vi "CPU_MEM_read_mem.vi"(11 "address":u16 format="%04x") -> (3 "value out":u8 format="%02x")   [LabVIEW 2018]
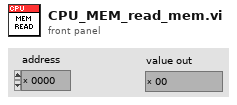
[diagram p1: front panel]
types:
  T1 = enum16{"init", "read DDR", "read PDR", "write DDR", "write PDR"}
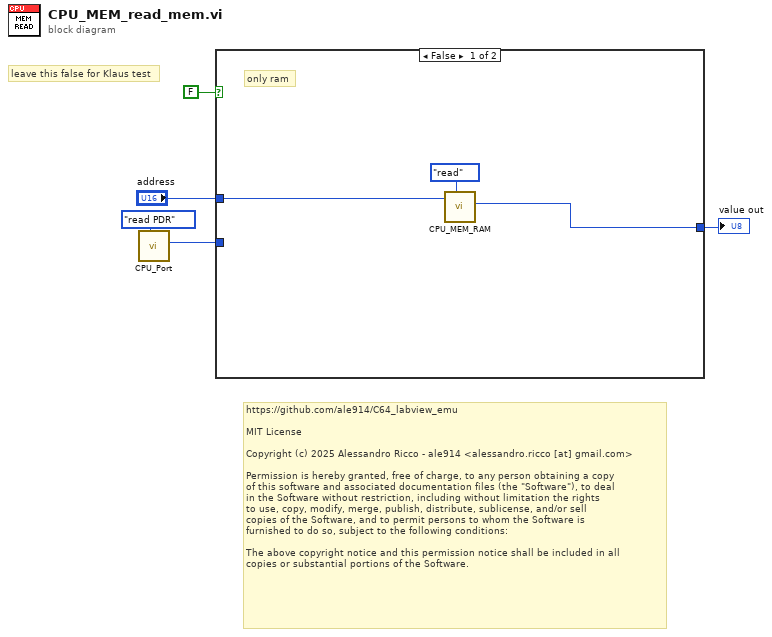
[diagram p0: block diagram]
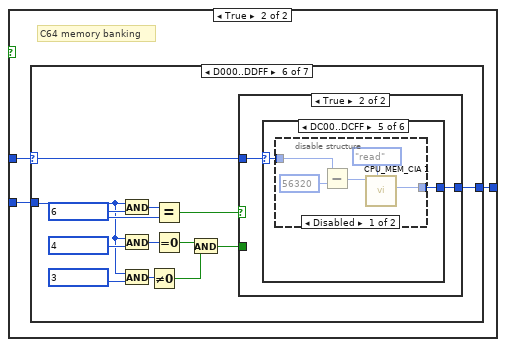
[diagram p2: hidden frame]
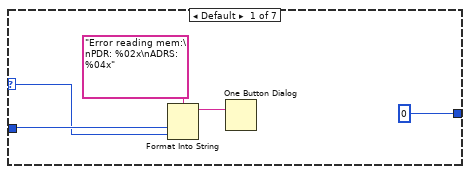
[diagram p3: hidden frame]
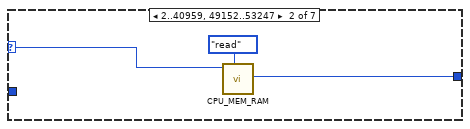
[diagram p4: hidden frame]
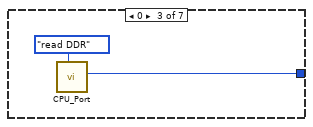
[diagram p5: hidden frame]
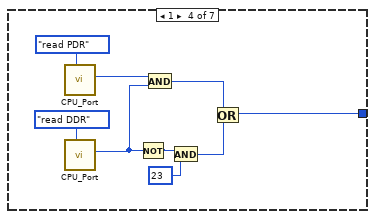
[diagram p6: hidden frame]
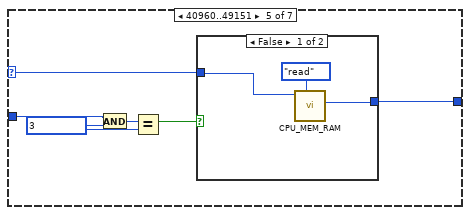
[diagram p7: hidden frame]
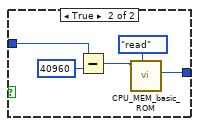
[diagram p8: hidden frame]
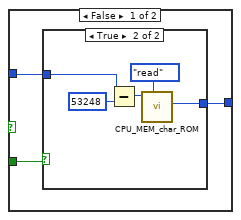
[diagram p9: hidden frame]
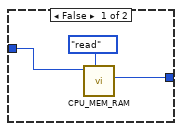
[diagram p10: hidden frame]
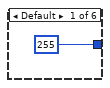
[diagram p11: hidden frame]
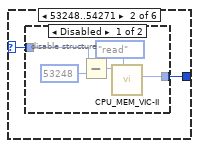
[diagram p12: hidden frame]
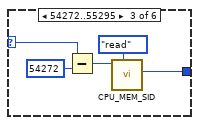
[diagram p14: hidden frame]
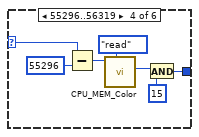
[diagram p15: hidden frame]
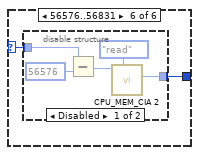
[diagram p17: hidden frame]
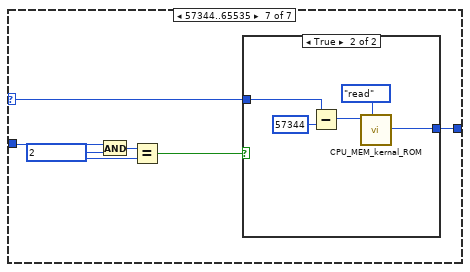
[diagram p19: hidden frame]
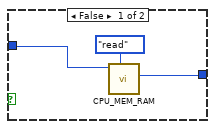
[diagram p20: hidden frame]
diagram:
  # "https://github.com/ale914/C64_labview_emu\n\nMIT License\n\nCopyright (c) 2025 Alessandro Ricco - ale914 <alessandro.ricco [at] gmail.com>\n\nPermission is hereby granted, free of charge, to any person obtaining a copy\nof this software and associated documentation files (the \"Software\"), to deal\nin the Software without restriction, including without limitation the rights\nto use, copy, modify, merge, publish, distribute, sublicense, and/or sell\ncopies of the Software, and to permit persons to whom the Software is\nfurnished to do so, subject to the following conditions:\n\nThe above copyright notice and this permission notice shall be included in all\ncopies or substantial portions of the Software."
  # "leave this false for Klaus test"
  n1 = call "CPU_Port.vi"("oper"=T1."read PDR") -> ("value out"=w2:u8)  [unwired: 10 in]
  n2 = case shown="False" FALSE {
    tunnel: "address" -> [w7 w11]
    tunnel: [w6 w10] -> w4
    tunnel: w2 -> [_ w9]
    frame False {
      # "only ram"
      n3 = call "CPU_MEM_RAM.vi"("oper"=enum16{"init", "read", "write"}."read", "address"=w7) -> ("value out"=w6:u8)  [unwired: 8 in, 1 out]
    }
    frame True {
      # "C64 memory banking"
      n4 = case shown="D000..DDFF" w11 {
        selector: w11 -> [w12 w17 _ _ w35 w54 w107]
        tunnel: [u8 0 ("value out") w18 w20 w25 w36 w55 w108] -> w10
        tunnel: w9 -> [w14 _ _ _ w34 w48 w106]
        frame Default {
          n5 = Format Into String(format string="Error reading mem:\nPDR: %02x\nADRS: %04x", w14, w12) -> (resulting string=w13:string)  [unwired: 2 in, 1 out]
          n6 = One Button Dialog(message=w13) -> ()  [unwired: 1 in, 1 out]
        }
        frame 2..40959, 49152..53247 {
          n7 = call "CPU_MEM_RAM.vi"("oper"=enum16{"init", "read", "write"}."read", "address"=w17) -> ("value out"=w18:u8)  [unwired: 8 in, 1 out]
        }
        frame 0 {
          n8 = call "CPU_Port.vi"("oper"=T1."read DDR") -> ("value out"=w20:u8)  [unwired: 10 in]
        }
        frame 1 {
          n9 = call "CPU_Port.vi"("oper"=T1."read PDR") -> ("value out"=w28:u8)  [unwired: 10 in]
          n10 = call "CPU_Port.vi"("oper"=T1."read DDR") -> ("value out"=w27:u8)  [unwired: 10 in]
          n11 = Not(x=w27) -> (.not. x?=w23:u8)
          n12 = And(x=w28, y=w27) -> (x .and. y?=w26:u8)
          n13 = And(x=w23, y=u8 23) -> (x .and. y?=w22:u8)
          n14 = Or(x=w26, y=w22) -> (x .or. y?=w25:u8)
        }
        frame 40960..49151 {
          w32 = u8 3 ("y")
          n15 = And(x=w34, y=w32) -> (x .and. y?=w33:u8)
          n16 = Equal?(x=w33, y=w32) -> (x = y?=w31:bool)
          n17 = case shown="False" w31 {
            tunnel: [w39 w43] -> w36
            tunnel: w35 -> [w37 w42]
            frame False {
              n18 = call "CPU_MEM_RAM.vi"("oper"=enum16{"init", "read", "write"}."read", "address"=w37) -> ("value out"=w39:u8)  [unwired: 8 in, 1 out]
            }
            frame True {
              n19 = Subtract(x=w42, y=u16 40960 ("address")) -> (x-y=w40:u16)
              n20 = call "CPU_MEM_basic_ROM.vi"("oper"=enum16{"init", "read", "write"}."read", "address"=w40) -> ("value out"=w43:u8)  [unwired: 8 in, 1 out]
            }
          }
        }
        frame 53248..56831 {
          w53 = u8 6 ("y")
          n21 = And(x=w48, y=w53) -> (x .and. y?=w57:u8)
          n22 = And(x=w48, y=u8 4) -> (x .and. y?=w51:u8)
          n23 = And(x=w48, y=u8 3) -> (x .and. y?=w47:u8)
          n24 = Not Equal To 0?(x=w47) -> (x != 0?=w46:bool)
          n25 = Equal?(x=w57, y=w53) -> (x = y?=w56:bool)
          n26 = Equal To 0?(x=w51) -> (x = 0?=w50:bool)
          n27 = And(x=w50, y=w46) -> (x .and. y?=w45:bool)
          n28 = case shown="True" w56 {
            tunnel: [w60 w69] -> w55
            tunnel: w54 -> [w59 w70]
            tunnel: w45 -> [w58 _]
            frame False {
              n29 = case shown="True" w58 {
                tunnel: [w63 w67] -> w60
                tunnel: w59 -> [w61 w64]
                frame False {
                  n30 = call "CPU_MEM_RAM.vi"("oper"=enum16{"init", "read", "write"}."read", "address"=w61) -> ("value out"=w63:u8)  [unwired: 8 in, 1 out]
                }
                frame True {
                  n31 = Subtract(x=w64, y=u16 53248 ("address")) -> (x-y=w65:u16)
                  n32 = call "CPU_MEM_char_ROM.vi"("oper"=enum16{"init", "read", "write"}."read", "address"=w65) -> ("value out"=w67:u8)  [unwired: 9 in]
                }
              }
            }
            frame True {
              n33 = case shown="DC00..DCFF" w70 {
                selector: w70 -> [_ w72 w80 w89 w91 w98]
                tunnel: [u8 255 ("value out") w73 w82 w84 w92 w99] -> w69
                frame Default {
                }
                frame 53248..54271 {
                  n34 = disable-structure shown="Disabled" {
                    disable-tunnel: [w77 _] -> w73
                    disable-tunnel: w72 -> [w75 _]
                    frame Disabled {
                      n35 = Subtract(x=w75, y=u16 53248 ("address")) -> (x-y=w74:u16)
                      n36 = call "CPU_MEM_VIC-II.vi"("oper"=enum16{"init", "read", "write"}."read", "address"=w74) -> ("value out"=w77:u8)  [unwired: 8 in, 1 out]
                    }
                    frame Enabled {
                    }
                  }
                }
                frame 54272..55295 {
                  n37 = Subtract(x=w80, y=u16 54272 ("address")) -> (x-y=w79:u16)
                  n38 = call "CPU_MEM_SID.vi"("oper"=enum16{"init", "read", "write"}."read", "address"=w79) -> ("value out"=w82:u8)  [unwired: 9 in]
                }
                frame 55296..56319 {
                  n39 = Subtract(x=w89, y=u16 55296 ("address")) -> (x-y=w88:u16)
                  n40 = call "CPU_MEM_Color.vi"("oper"=enum16{"init", "read", "write"}."read", "address"=w88) -> ("value out"=w86:u8)  [unwired: 8 in, 1 out]
                  n41 = And(x=w86, y=u8 15 ("address")) -> (x .and. y?=w84:u8)
                }
                frame 56320..56575 {
                  n42 = disable-structure shown="Disabled" {
                    disable-tunnel: [w96 _] -> w92
                    disable-tunnel: w91 -> [w94 _]
                    frame Disabled {
                      n43 = Subtract(x=w94, y=u16 56320 ("address")) -> (x-y=w93:u16)
                      n44 = call "CPU_MEM_CIA 1.vi"("oper"=enum16{"init", "read", "write"}."read", "address"=w93) -> ("value out"=w96:u8)  [unwired: 8 in, 1 out]
                    }
                    frame Enabled {
                    }
                  }
                }
                frame 56576..56831 {
                  n45 = disable-structure shown="Disabled" {
                    disable-tunnel: [w103 _] -> w99
                    disable-tunnel: w98 -> [w101 _]
                    frame Disabled {
                      n46 = Subtract(x=w101, y=u16 56576 ("address")) -> (x-y=w100:u16)
                      n47 = call "CPU_MEM_CIA 2.vi"("oper"=enum16{"init", "read", "write"}."read", "address"=w100) -> ("value out"=w103:u8)  [unwired: 9 in]
                    }
                    frame Enabled {
                    }
                  }
                }
              }
            }
          }
        }
        frame 57344..65535 {
          w105 = u8 2 ("y")
          n48 = And(x=w106, y=w105) -> (x .and. y?=w110:u8)
          n49 = Equal?(x=w110, y=w105) -> (x = y?=w109:bool)
          n50 = case shown="True" w109 {
            tunnel: [w113 w117] -> w108
            tunnel: w107 -> [w111 w115]
            frame False {
              n51 = call "CPU_MEM_RAM.vi"("oper"=enum16{"init", "read", "write"}."read", "address"=w111) -> ("value out"=w113:u8)  [unwired: 8 in, 1 out]
            }
            frame True {
              n52 = Subtract(x=w115, y=u16 57344 ("address")) -> (x-y=w114:u16)
              n53 = call "CPU_MEM_kernal_ROM.vi"("oper"=enum16{"init", "read", "write"}."read", "address"=w114) -> ("value out"=w117:u8)  [unwired: 8 in, 1 out]
            }
          }
        }
      }
    }
  }
  "value out" <- w4
